vi "ScaleTraj.vi"(10 "ScalingCoef":dbl=1.0, 11 "Averaged Gait":dbl[][](array[numeric])) -> (2 "ScaledGait":dbl[][](array[numeric]), 3 "XY Graph":cluster{"Y":dbl[], "Y":dbl[]}[](graph))   [LabVIEW 2015]
uses:
  <userlib>/_OpenG.lib/array/array.llb/Index 1D Array Elements (DBL)__ogtk.vi
  <vilib>/imath/engines/lvmath2/RunTimeEngine/IndexRead/NIMS V(S).vi
  <instcachedir>/0/NIMS V(S)_0488751826AF41519A22953C041130DC.lvgen/NIMS V(S)_0488751826AF41519A22953C041130DC_000.vi
  <vilib>/imathl/engines/lvmath/Functions/Error Handling/Create Error.vi
  <vilib>/imath/engines/lvmath2/RunTimeEngine/ArithmeticOperatorToken/NIMS_ArithmeticOperator_power(S).vi
  <instcachedir>/0/NIMS_ArithmeticOperator_power(S)_DFB67823F1414E5097C86E39787D8CA8.lvgen/NIMS_ArithmeticOperator_power(S)_DFB67823F1414E5097C86E39787D8CA8_015.vi
  <instcachedir>/0/NIMS_ArithmeticOperator_power(S)_DFB67823F1414E5097C86E39787D8CA8.lvgen/NIMS_ArithmeticOperator_power(S)_DFB67823F1414E5097C86E39787D8CA8_014.vi
  <vilib>/imath/engines/lvmath2/RunTimeEngine/ErrorHandling/NIMS_Create Error From Enums.vi
  <vilib>/imath/engines/lvmath2/RunTimeEngine/NodeEndStatement/NIMS_NodeEndStatement_Output.vi
  <instcachedir>/0/NIMS_NodeEndStatement_Output_53EC0D466D134D7ABD903AC30B43404B.lvgen/NIMS_NodeEndStatement_Output_53EC0D466D134D7ABD903AC30B43404B_005.vi
  <vilib>/imath/engines/lvmath2/RunTimeEngine/ErrorHandling/NIMS_Finalize Error.vi
panel:
  out "XY Graph 2":cluster{dbl[], "yi":dbl[]}(graph)
  out "XY":cluster{"Mean":dbl[], "Mean":dbl[]}[](array[cluster])
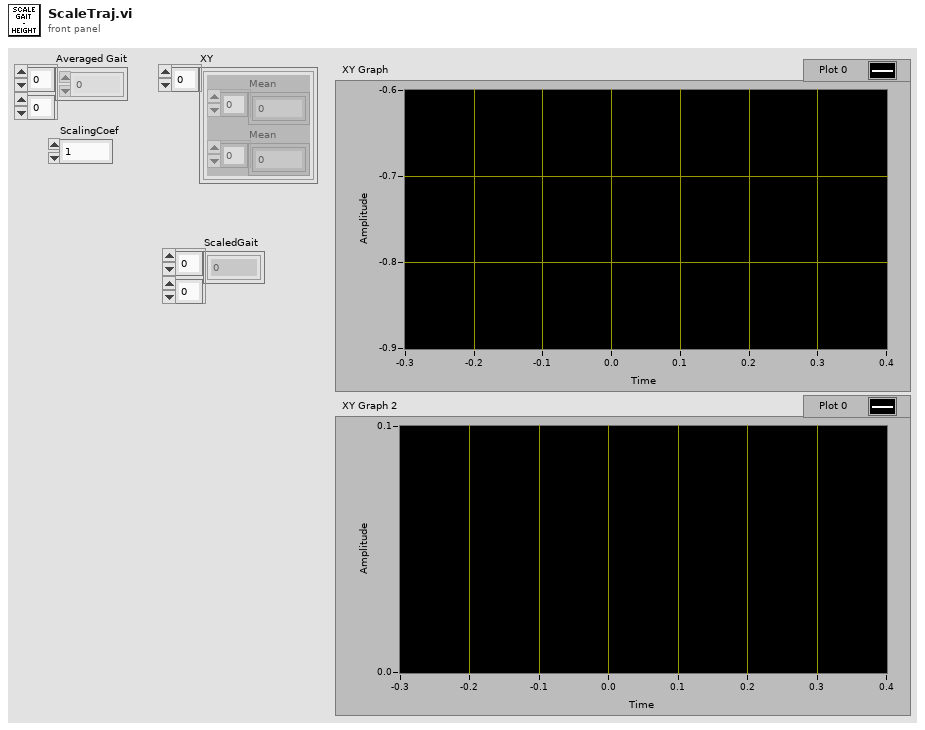
[diagram p1: front panel]
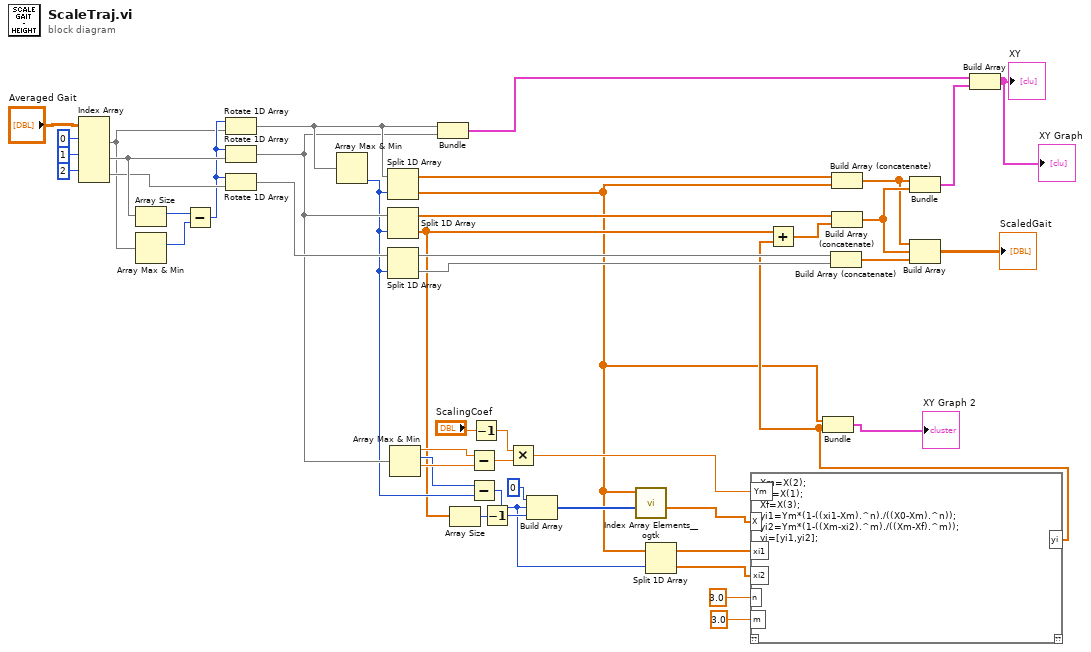
[diagram p0: block diagram]
diagram:
  n1 = Index Array(array="Averaged Gait", index (row) #1=0 ("index (row)"), index (row) #2=1 ("index (row)"), index (row) #3=2 ("index (row)")) -> (element #1=w34:dbl[], element #2=w43:dbl[], element #3=w39:dbl[])  [unwired: 3 in]
  n2 = Array Size(array=w43) -> (size(s)=w42:i32)
  n3 = Array Max & Min(array=w34) -> (max index (indices)=w41:i32)  [unwired: 3 out]
  n4 = Subtract(x=w42, y=w41) -> (x-y=w38:i32)
  n5 = Rotate 1D Array(1:w34, 2:w38) -> (0:w36:dbl[])
  n6 = Rotate 1D Array(1:w43, 2:w38) -> (0:w31:dbl[])
  n7 = Rotate 1D Array(1:w39, 2:w38) -> (0:w35:dbl[])
  n8 = Array Max & Min(array=w36) -> (min index (indices)=w17:i32)  [unwired: 3 out]
  n9 = Split 1D Array(array=w36, index=w17) -> (first subarray=w26:dbl[], second subarray=w6:dbl[])
  n10 = Split 1D Array(array=w31, index=w17) -> (first subarray=w27:dbl[], second subarray=w13:dbl[])
  n11 = Split 1D Array(array=w35, index=w17) -> (first subarray=w25:dbl[], second subarray=w24:dbl[])
  n12 = Array Max & Min(array=w31) -> (max value=w29:dbl, max index (indices)=w18:i32, min value=w30:dbl)  [unwired: 1 out]
  n13 = Bundle(w36, w31) -> (w47:cluster{dbl[], dbl[]})  [unwired: 1 in]
  n14 = Array Size(array=w13) -> (size(s)=w33:i32)
  n15 = Subtract(x=w29, y=w30) -> (x-y=w15:dbl)
  n16 = Subtract(x=w18, y=w17) -> (x-y=w5:i32)
  n17 = Decrement(x="ScalingCoef") -> (x-1=w14:dbl)
  n18 = Decrement(x=w33) -> (x-1=w16:i32)
  n19 = Multiply(x=w14, y=w15) -> (x*y=w10:dbl)
  n20 = Build Array(0 ("element"), w5, w16) -> (w11:i32[])
  n21 = call-poly <userlib>:"Index Array Elements__ogtk.vi"("indices"=w11, "array"=w6) -> ("elements"=w9:dbl[])  [unwired: 9 in]
  n22 = Split 1D Array(array=w6, index=w5) -> (first subarray=w4:dbl[], second subarray=w3:dbl[])
  n23 = mathscript code="Xm=X(2);\nX0=X(1);\nXf=X(3);\nyi1=Ym*(1-((xi1-Xm).^n)./((X0-Xm).^n));\nyi2=Ym*(1-((Xm-xi2).^m)./((Xm-Xf).^m));\nyi=[yi1,yi2];"("Ym"=w10, "X"=w9, "xi1"=w4, "n"=3.0 ("element"), "xi2"=w3, "m"=3.0 ("element")) -> ("yi"=w7:dbl[])  [unwired: 1 in, 1 out]
  n24 = Add(x=w13, y=w7) -> (x+y=w28:dbl[])
  n25 = Bundle(w6, "yi"=w7) -> (→"XY Graph 2":cluster{dbl[], "yi":dbl[]})  [unwired: 1 in]
  n26 = Build Array (concatenate)(w25, w24) -> (w22:dbl[])
  n27 = Build Array (concatenate)(w26, w6) -> (w20:dbl[])
  n28 = Build Array (concatenate)(w27, w28) -> (w21:dbl[])
  n29 = Bundle(w20, w21) -> (w23:cluster{dbl[], dbl[]})  [unwired: 1 in]
  n30 = Build Array(w20, w21, w22) -> (→"ScaledGait":dbl[][])
  n31 = Build Array(w47, w23) -> (→"XY" →"XY Graph":cluster{dbl[], dbl[]}[])
